vi "Validate Gear Position.vi"(9 "Error Limit [Degrees]":dbl=5.0, 10 "Simulated Gear Position [Degrees]":dbl, 11 "Real Gear Position [Degrees]":dbl) -> (3 "Valid":bool)   [LabVIEW 2018]
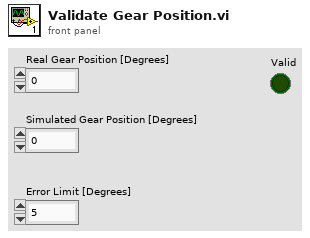
[diagram p1: front panel]
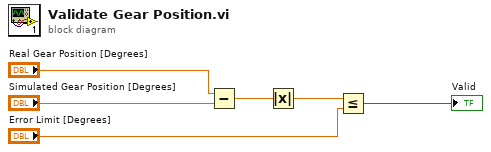
[diagram p0: block diagram]
diagram:
  n1 = Subtract(x="Real Gear Position [Degrees]", y="Simulated Gear Position [Degrees]") -> (x-y=w4:dbl)
  n2 = Absolute Value(x=w4) -> (abs(x)=w3:dbl)
  n3 = Less Or Equal?(x=w3, y="Error Limit [Degrees]") -> (x <= y?=→"Valid":bool)
